vi "_Parse Markdown Control Elements.vi"(8 "Error in":errorcluster caption="Error in (no error)", 11 "Lines":string[](array[string])) -> (0 "Error out":errorcluster, 2 "Array":T1[](array[typedef]), 3 "Lines (dup)":string[](array[string]))   [LabVIEW 2017, in "csmdoc.lvlib"]
uses:
  csmdoc.lvlib
  _Typedef/DocNote.ctl
  _tool/_file/csm-file-support.lvlib
  Communicable State Machine.lvlib
  _Shared/CSM Shared.lvlib
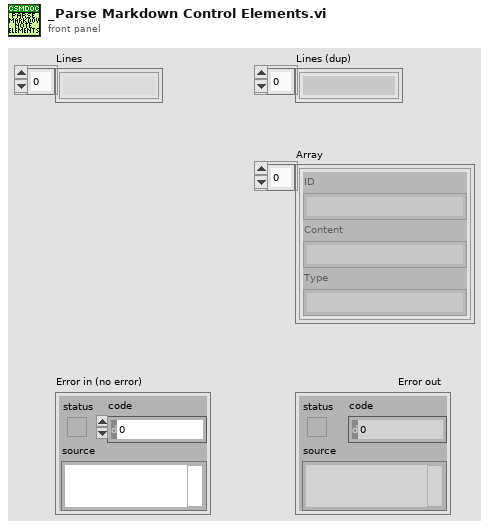
[diagram p1: front panel]
types:
  T1 = typedef "csmdoc.lvlib/DocNote.ctl" = cluster{"ID":string, "Content":string, "Type":string}
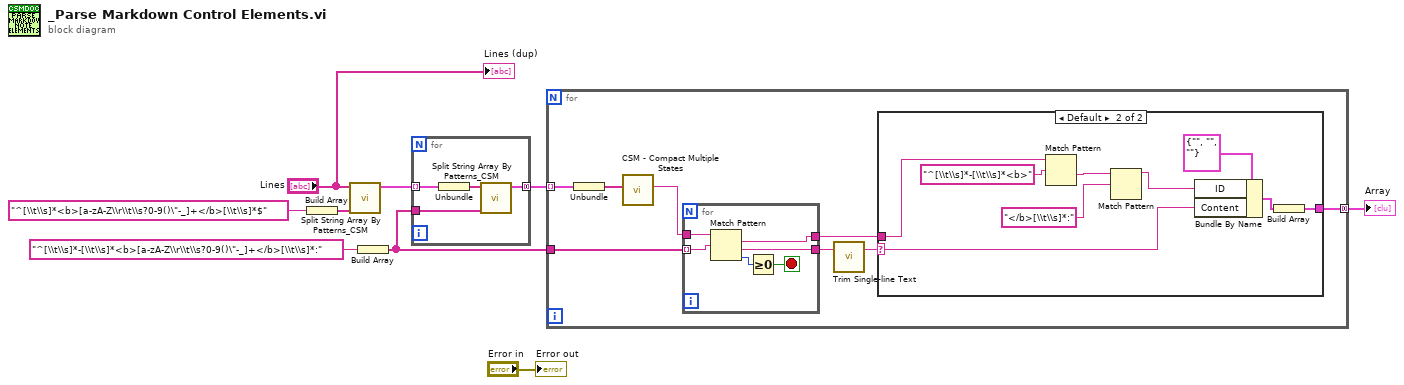
[diagram p0: block diagram]
diagram:
  n1 = Build Array("^[\\t\\s]*<b>[a-zA-Z\\r\\t\\s?0-9()\"-_]+</b>[\\t\\s]*$" ("delimited string")) -> (w4:string[])
  n2 = call "Split String Array By Patterns_CSM.vi"("Patterns"=w4, "Text Array"="Lines") -> ("Array"=w5:cluster{"filtered array":string[]}[])  [unwired: 9 in]
  n3 = Build Array("^[\\t\\s]*-[\\t\\s]*<b>[a-zA-Z\\r\\t\\s?0-9()\"-_]+</b>[\\t\\s]*:" ("delimited string")) -> (w8:string[])
  n4 = for {
    tunnel: w5 -> [w13] mode=indexing
    tunnel: [w11] -> w6 mode=concatenating
    tunnel: w8 -> [w10]
    n5 = Unbundle(w13) -> ("filtered array"=w12:string[])
    n6 = call "Split String Array By Patterns_CSM.vi"("Patterns"=w10, "Text Array"=w12) -> ("Array"=w11:cluster{"filtered array":string[]}[])  [unwired: 9 in]
  }
  n7 = for {
    tunnel: w6 -> [w21] mode=indexing
    tunnel: [w18] -> w9 mode=concatenating
    tunnel: w8 -> [w17]
    n8 = Unbundle(w21) -> ("filtered array"=w15:string[])
    n9 = call "CSM - Compact Multiple States.vi"("Multiple States"=w15) -> ("States"=w14:string)  [unwired: 9 in]
    n10 = for {
      tunnel: w14 -> [w26]
      tunnel: [w27] -> w20
      tunnel: w17 -> [w25] mode=indexing
      tunnel: [w22] -> w16
      stop <- w23 stop-if-true
      n11 = Match Pattern(string=w26, regular expression=w25) -> (match substring=w22:string, after substring=w27:string, offset past match=w24:i32)  [unwired: 1 in, 1 out]
      n12 = Greater Or Equal To 0?(x=w24) -> (x >= 0?=w23:bool)
    }
    n13 = call "Trim Single-line Text.vi"("single-line text"=w20) -> ("trimed text"=w19:string)  [unwired: 2 in]
    n14 = case shown="Default" w19 {
      selector: w19 -> [_ w33]
      tunnel: [_ w34] -> w18
      tunnel: w16 -> [_ w29]
      frame "" {
      }
      frame Default {
        n15 = Match Pattern(string=w29, regular expression="^[\\t\\s]*-[\\t\\s]*<b>") -> (after substring=w32:string)  [unwired: 1 in, 3 out]
        n16 = Match Pattern(string=w32, regular expression="</b>[\\t\\s]*:" ("delimited string")) -> (before substring=w28:string)  [unwired: 1 in, 3 out]
        n17 = Bundle By Name(cluster=T1 {"ID"="", "Content"="", "Type"=""} ("Cluster"), "ID"=w28, "Content"=w33) -> (w35:T1)
        n18 = Build Array(w35) -> (w34:T1[])
      }
    }
  }
  "Array" <- w9
  "Error out" <- "Error in"
  "Lines (dup)" <- "Lines"
